vi "Draw More Options Icon.vi"(8 "error in (no error)":errorcluster, 10 "Index To Add":i32, 11 "Toolbar Control in":refnum<class "Toolbar Control.lvclass">) -> (0 "error out":errorcluster, 2 "More Options Image":picture, 3 "Toolbar Control out":refnum<class "Toolbar Control.lvclass">)   [LabVIEW 2011, in "Toolbar Control.lvclass"]
doc: "This VI will create the <B>More Options Image</B>, and add it at <B>Index To Add</B>.\n\n-------------\nDeveloped by Brian Hoover (hooovahh)"
uses:
  Toolbar Control.lvclass
  Toolbar Control.lvclass/Toolbar Control.ctl
  Controls/Mouse State.ctl
  Controls/Horizontal Initialize Settings.ctl
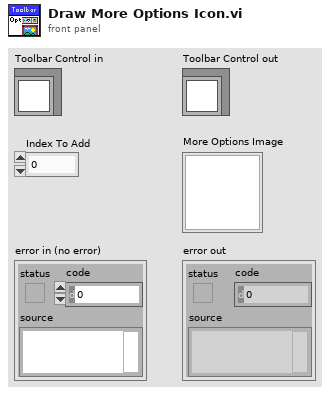
[diagram p1: front panel]
types:
  T1 = typedef "Horizontal Initialize Settings.ctl" = cluster{"Button Width":i32, "Button Height":i32, "Separator Width":i32, "More Options Width":i32}
  T2 = typedef "Mouse State.ctl" = enum8{"Normal", "Mouse Over", "Mouse Down"}
  T3 = typedef "LVRectTypeDef.ctl" = cluster{"Left":i16, "Top":i16, "Right":i16, "Bottom":i16}
  T4 = typedef "Toolbar Control.lvclass/Icon Data.ctl" = cluster{"Original Image Path":path, "Original Image Data":T5, "Scaled Icon":picture, "Button Name":string, "Button State":T6, "Icon Type":T7}
  T5 = typedef "imagedata.ctl" = cluster{"image type":i32, "image depth":i32, "image":u8[], "mask":u8[], "colors":u32[], "Rectangle":cluster{"left":i16, "top":i16, "right":i16, "bottom":i16}}
  T6 = typedef "Toolbar Control.lvclass/Button State.ctl" = enum8{"Enabled", "Disabled", "Disabled and Grayed Out"}
  T7 = typedef "Icon Type.ctl" = enum16{"Normal Icon", "Separator Icon", "More Options"}
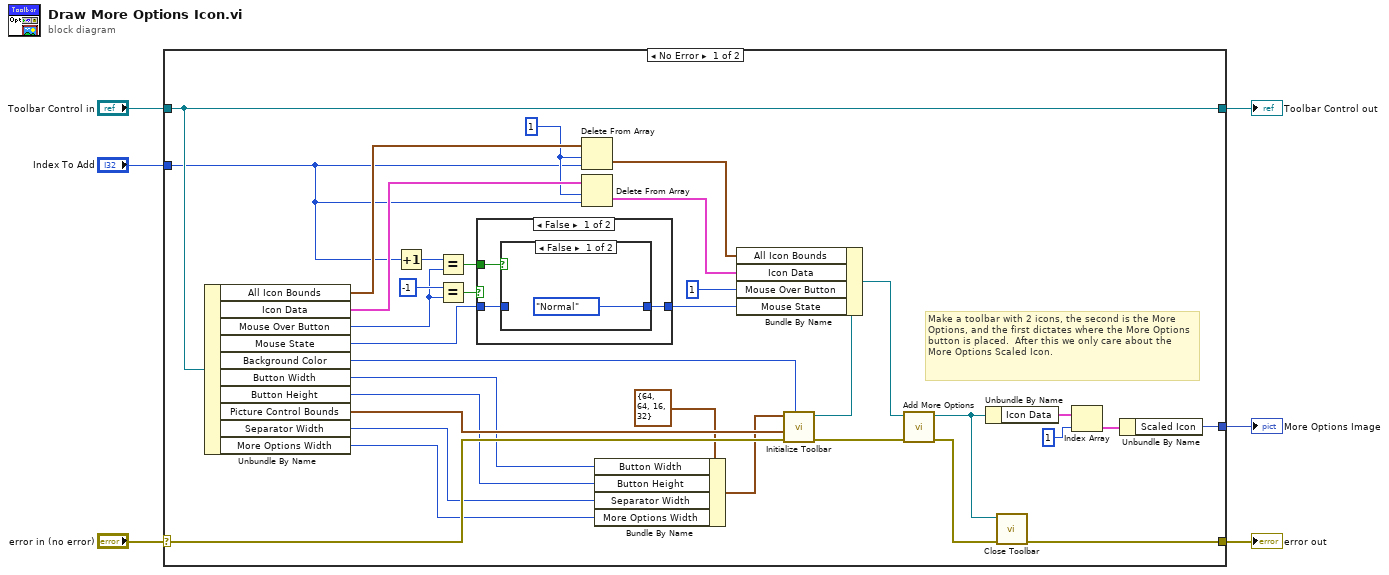
[diagram p0: block diagram]
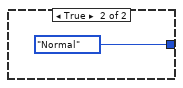
[diagram p3: hidden frame]
diagram:
  n1 = case shown="No Error" "error in (no error)" {
    selector: "error in (no error)" -> [w22 w48]
    tunnel: [w14 w48] -> w5
    tunnel: [w40 w47] -> w3
    tunnel: "Toolbar Control in" -> [w40 w47]
    tunnel: [w21 _] -> w2
    tunnel: "Index To Add" -> [w18 _]
    frame No Error {
      w20 = 1 ("length")
      # "Make a toolbar with 2 icons, the second is the More Options, and the first dictates where the More Options button is placed.  After this we only care about the More Options Scaled Icon."
      n2 = Unbundle By Name(w40) -> ("All Icon Bounds"=w26:T3[], "Icon Data"=w27:T4[], "Mouse Over Button"=w19:i32, "Mouse State"=w32:T2, "Background Color"=w39:u32, "Button Width"=w7:i32, "Button Height"=w10:i32, "Picture Control Bounds"=w38:T3, "Separator Width"=w9:i32, "More Options Width"=w8:i32)
      n3 = Increment(x=w18) -> (x+1=w16:i32)
      n4 = Equal?(x=w16, y=w19) -> (x = y?=w17:bool)
      n5 = Equal?(x=-1, y=w19) -> (x = y?=w31:bool)
      n6 = case shown="False" w31 {
        tunnel: w32 -> [w43 _]
        tunnel: [w41 Mouse_State."Normal" ("Mouse State")] -> w30
        tunnel: w17 -> [w42 _]
        frame False {
          n7 = case shown="False" w42 {
            tunnel: w43 -> [_ w45]
            tunnel: [Mouse_State."Normal" ("Mouse State") w45] -> w41
            frame False {
            }
            frame True {
            }
          }
        }
        frame True {
        }
      }
      n8 = Delete From Array(array=w26, length=w20, index=w18) -> (deleted portion=w24:T3[])  [unwired: 1 out]
      n9 = Delete From Array(array=w27, length=w20, index=w18) -> (deleted portion=w25:T4[])  [unwired: 1 out]
      n10 = Bundle By Name(cluster=T1 {"Button Width"=64, "Button Height"=64, "Separator Width"=16, "More Options Width"=32} ("Horizontal Icon Settings"), "Button Width"=w7, "Button Height"=w10, "Separator Width"=w9, "More Options Width"=w8) -> (w11:T1)
      n11 = call "Initialize Toolbar.vi"("Background Color"=w39, "error in (no error)"=w22, "Picture Control Bounds"=w38, "Horizontal Icon Settings"=w11) -> ("error out"=w36:errorcluster, "Toolbar Control out"=w37:refnum<class "Toolbar Control.lvclass">)  [unwired: 6 in]
      n12 = Bundle By Name(cluster=w37, "All Icon Bounds"=w24, "Icon Data"=w25, "Mouse Over Button"=1, "Mouse State"=w30) -> (w35:refnum<class "Toolbar Control.lvclass">)
      n13 = call "Add More Options.vi"("error in (no error)"=w36, "Toolbar Control in"=w35) -> ("error out"=w15:errorcluster, "Toolbar Control out"=w13:refnum<class "Toolbar Control.lvclass">)  [unwired: 8 in]
      n14 = Unbundle By Name(w13) -> ("Icon Data"=w29:T4[])
      n15 = call "Close Toolbar.vi"("error in (no error)"=w15, "Toolbar Control in"=w13) -> ("error out"=w14:errorcluster)  [unwired: 9 in]
      n16 = Index Array(array=w29, index=1) -> (element=w28:T4)
      n17 = Unbundle By Name(w28) -> ("Scaled Icon"=w21:picture)
    }
    frame Error {
    }
  }
  "error out" <- w5
  "Toolbar Control out" <- w3
  "More Options Image" <- w2
